vi "Odometry.vi"() -> ()   [LabVIEW 2019]
uses:
  <vilib>/myRIO/Common/Instrument Driver Framework/myRIO v1.0/Encoder/typedefs/Encoder Signal Mode.ctl
  <vilib>/myRIO/Instrument Drivers/Onboard IO/Encoder/typedefs/Encoder Reference.ctl
  <vilib>/myRIO/Common/Instrument Driver Framework/Utilities/typedefs/myRIO Generic Hardware Reference.ctl
  <vilib>/myRIO/Common/Instrument Driver Framework/Utilities/typedefs/Hardware Version Enum.ctl
  <vilib>/myRIO/Common/Instrument Driver Framework/Utilities/typedefs/myRIO v1.0 Reference.ctl
  <vilib>/myRIO/Common/Instrument Driver Framework/Utilities/typedefs/Generic FPGA Reference.ctl
  <vilib>/myRIO/Common/Instrument Driver Framework/myRIO v1.0/Encoder/typedefs/Encoder Channels Enum.ctl
  <vilib>/myRIO/Common/Instrument Driver Framework/myRIO v1.0/Encoder/typedefs/Encoder Configuration v1.0.ctl
  <vilib>/userDefined/High Color/nirio_resource_hc.ctl
  <vilib>/Platform/TimedLoop/XDataNode/timing_clust.ctl
  <vilib>/Platform/TimedLoop/XDataNode/nitl_modes.ctl
  <vilib>/Platform/TimedLoop/XDataNode/wakeup.ctl
  <vilib>/myRIO/Instrument Drivers/Onboard IO/PWM/typedefs/PWM Reference.ctl
  <vilib>/myRIO/Common/Instrument Driver Framework/myRIO v1.0/PWM/typedefs/PWM Channels Enum.ctl
  <vilib>/myRIO/Instrument Drivers/Onboard IO/PWM/typedefs/PWM Configuration.ctl
  <vilib>/myRIO/Instrument Drivers/Onboard IO/DIO/typedefs/DIO Reference.ctl
  <vilib>/myRIO/Common/Instrument Driver Framework/myRIO v1.0/DIO/typedefs/DIO Channels List.ctl
  <vilib>/myRIO/Common/Instrument Driver Framework/myRIO v1.0/DIO/typedefs/DIO Channels Enum.ctl
  <vilib>/myRIO/Common/Instrument Driver Framework/Utilities/vis/Is FPGA Ref Available.vi
  <vilib>/myRIO/Common/Instrument Driver Framework/myRIO v1.0/Encoder/vis/myRIO v1.1 Open Encoder.vi
  <vilib>/myRIO/Instrument Drivers/Onboard IO/Encoder/vis/Read.vi
  <vilib>/myRIO/Common/Instrument Driver Framework/myRIO v1.0/PWM/vis/myRIO v1.1 Open PWM.vi
  <vilib>/myRIO/Instrument Drivers/Onboard IO/PWM/vis/Set Duty Cycle and Frequency.vi
  <vilib>/myRIO/Common/Instrument Driver Framework/myRIO v1.0/DIO/vis/myRIO v1.1 Open DIO.vi
  <vilib>/myRIO/Instrument Drivers/Onboard IO/DIO/vis/Write.vi
  <vilib>/myRIO/Common/Instrument Driver Framework/Utilities/vis/Validate Channels.vi
  <vilib>/myRIO/Common/Instrument Driver Framework/myRIO v1.0/Encoder/vis/myRIO v1.0 Reserve Encoder.vi
  <vilib>/myRIO/Common/Instrument Driver Framework/myRIO v1.0/PWM/vis/myRIO v1.0 Reserve PWM.vi
  <vilib>/myRIO/Common/Instrument Driver Framework/myRIO v1.0/DIO/vis/myRIO v1.0 Reserve DIO.vi
  <vilib>/myRIO/Common/Instrument Driver Framework/myRIO v1.0/Encoder/vis/myRIO v1.0 Build MUX Configuration Encoder.vi
  <vilib>/myRIO/Common/Instrument Driver Framework/myRIO v1.0/Resource Manager/vis/myRIO v1.0 Reserve Channel List.vi
  <vilib>/myRIO/Common/Instrument Driver Framework/myRIO v1.0/PWM/vis/myRIO v1.0 Build MUX Configuration PWM.vi
  <vilib>/myRIO/Common/Instrument Driver Framework/myRIO v1.0/DIO/vis/myRIO v1.0 Build MUX Configuration DIO.vi
  <vilib>/myRIO/Common/Instrument Driver Framework/myRIO v1.0/Resource Manager/vis/myRIO v1.0 Create Configuration List.vi
  <vilib>/myRIO/Common/Instrument Driver Framework/myRIO v1.0/Resource Manager/vis/myRIO v1.0 Reserve Channel.vi
  <vilib>/myRIO/Common/Instrument Driver Framework/myRIO v1.0/Resource Manager/vis/myRIO v1.0 Unreserve Channel.vi
  <vilib>/myRIO/Common/Instrument Driver Framework/myRIO v1.0/Resource Manager/vis/myRIO v1.0 Build Mutex Name.vi
  <vilib>/Utility/VariantDataType/GetNumericInfo.vi
  <vilib>/Utility/error.llb/Error Cluster From Error Code.vi
  <vilib>/myRIO/Common/Instrument Driver Framework/myRIO v1.0/myRIO v1.1 Open.vi
  <vilib>/myRIO/Common/Instrument Driver Framework/Utilities/vis/IO Manager.vi
  <vilib>/myRIO/Common/Instrument Driver Framework/Utilities/vis/Configuration Manager.vi
  <vilib>/myRIO/Common/Instrument Driver Framework/myRIO v1.0/Resource Manager/vis/myRIO v1.0 Configure IO.vi
  <vilib>/myRIO/Common/Instrument Driver Framework/myRIO v1.0/myRIO v1.0 Close.vi
  <vilib>/myRIO/Common/Instrument Driver Framework/myRIO v1.0/Encoder/vis/myRIO v1.0 Configure Encoder.vi
  <vilib>/myRIO/Common/Instrument Driver Framework/myRIO v1.0/Encoder/vis/myRIO v1.0 Read Encoder.vi
  <vilib>/imath/engines/lvmath2/RunTimeEngine/NodeEndStatement/NIMS_NodeEndStatement_Output.vi
  <instcachedir>/0/NIMS_NodeEndStatement_Output_53EC0D466D134D7ABD903AC30B43404B.lvgen/NIMS_NodeEndStatement_Output_53EC0D466D134D7ABD903AC30B43404B_001.vi
  <vilib>/imath/engines/lvmath2/RunTimeEngine/ErrorHandling/NIMS_Finalize Error.vi
  <vilib>/myRIO/Common/Instrument Driver Framework/myRIO v1.0/PWM/vis/myRIO v1.0 Write PWM.vi
  <vilib>/myRIO/Common/Instrument Driver Framework/myRIO v1.0/DIO/vis/myRIO v1.0 Write DIO.vi
  <vilib>/imath/engines/lvmath2/RunTimeEngine/Managers/WorkSpace/UID Generator.vi
  <vilib>/imath/engines/lvmath2/RunTimeEngine/RunTimeType/NIMS_RunTimeType_From StrictType (excl LVString).vi
  <instcachedir>/0/NIMS_RunTimeType_From StrictType (excl LVString)_D8AFBA86A94845AAA577C895450664BD.lvgen/NIMS_RunTimeType_From StrictType (excl LVString)_D8AFBA86A94845AAA577C895450664BD_000.vi
  <vilib>/imath/engines/lvmath2/RunTimeEngine/LocalVariableDefStatement/MC_LocalVariableDefStatement_Display.vi
  <vilib>/imath/engines/lvmath2/RunTimeEngine/Managers/SymbolTable/Clear UID.vi
  <vilib>/myRIO/Express VI/Onboard IO/Encoder/Encoder Express VI.xnode
  <vilib>/myRIO/Instrument Drivers/Onboard IO/Encoder/vis/myRIO Encoder Open.xnode
  <vilib>/myRIO/Common/Instrument Driver Framework/myRIO v1.0/Encoder/typedefs/Encoder Count Direction Enum.ctl
  <vilib>/platform/TimedLoop/XDataNode/XDataNode.xnode
  <vilib>/myRIO/Express VI/Onboard IO/PWM/PWM Express VI.xnode
  <vilib>/myRIO/Instrument Drivers/Onboard IO/PWM/vis/myRIO PWM Open.xnode
  <vilib>/myRIO/Express VI/Onboard IO/DO/DO Express VI.xnode
  <vilib>/myRIO/Instrument Drivers/Onboard IO/DIO/vis/myRIO DIO Open.xnode
  <vilib>/Platform/TimedLoop/XDataNode/XDNodeRunTimeDep.lvlib
  <vilib>/myRIO/Instrument Drivers/Onboard IO/DIO/DIO.lvlib
  <vilib>/myRIO/Instrument Drivers/Onboard IO/Encoder/Encoder.lvlib
  <vilib>/myRIO/Instrument Drivers/Onboard IO/PWM/PWM.lvlib
  <vilib>/imath/engines/lvmath2/RunTimeEngine/Managers/SymbolTable/NIMS_WorkSpace.lvlib
panel:
  out "phiR chart case1":dynamicdata(graph)
  out "omegaR chart case1":dynamicdata(graph)
  in  "Tab Control":enum32{"Page 1", "Page 2", "Page 3"}(tab)
  out "XY Graph":cluster{"X":dbl, "Y":dbl}[](graph)
  in  "t1":dbl
  in  "t2":dbl
  in  "t3":dbl
  in  "Vmax (m/s)":dbl
  out "omega R now, desired case1":cluster{dbl, "omegaR":dbl}(graph)
  out "CarOmega case1":cluster{"actCarOmega":dbl, "desCarOmega":dbl}(graph)
  out "CarV case1":cluster{"actCarV":dbl, "desCarV":dbl}(graph)
  out "omega L now, desired case1":cluster{dbl, "omegaL":dbl}(graph)
  out "carV chart case1":dynamicdata(graph)
  out "omegaR":dbl
  out "omegaL":dbl
  in  "Stop case1":bool
  in  "Frequency R [Hz] case1":dbl=1000.0
  out "Duty R case1":dbl
  out "Duty L case1":dbl
  in  "Frequency L [Hz] case1":dbl=1000.0
  out "phiR":dbl
  out "phiL":dbl
  in  "R Gain":T1
  in  "L Gain":T1
  out "Encoder R":i32
  out "desPhiR":dbl
  out "CarOmega case2":cluster{"actCarOmega":dbl, "desCarOmega":dbl}(graph)
  out "CarV case2":cluster{"actCarV":dbl, "desCarV":dbl}(graph)
  in  "t5 case2":dbl
  in  "t6 case2":dbl
  in  "t7 case2":dbl
  in  "t8 case2":dbl
  in  "t9 case2":dbl
  in  "stop case2":bool
  in  "t4 case2":dbl
  out "Duty L case2":dbl
  in  "Frequency L [Hz] case2":dbl=1000.0
  out "phi L now, desired case2":cluster{dbl, "omegaL":dbl}(graph)
  out "phi R now, desired case2":cluster{dbl, "omegaR":dbl}(graph)
  in  "Vmax (m/s) case2":dbl
  in  "t1 case2":dbl
  in  "t2 case2":dbl
  in  "t3 case2":dbl
  in  "thetaDotmax case2":dbl
  out "carVTest Chart case2":dynamicdata(graph)
  out "XY Graph case2":dbl[][](graph)
  out "thetaDot case2":dbl
  out "carOmegaTest case2":dynamicdata(graph)
  in  "Frequency R [Hz] case2":dbl=1000.0
  out "Duty R case2":dbl
  in  "R Gain case2":T1
  in  "L Gain case2":T1
  in  "thetaDotmax case3":dbl
  in  "t7 case3":dbl
  in  "t6 case3":dbl
  in  "t5 case3":dbl
  in  "t4 case3":dbl
  in  "t3 case3":dbl
  in  "t2 case3":dbl
  in  "t1 case3":dbl
  out "thetaDot case3":dbl
  in  "Vmax (m/s) case3":dbl
  in  "stop case3":bool
  out "Duty R case3":dbl
  in  "Frequency R [Hz] case3":dbl=1000.0
  in  "Frequency L [Hz] case3":dbl=1000.0
  out "Duty L case3":dbl
  out "XY Graph case3":dbl[][](graph)
  out "phi L now, desired case3":cluster{dbl, "omegaL":dbl}(graph)
  out "CarV case3":cluster{"actCarV":dbl, "desCarV":dbl}(graph)
  out "CarOmega case3":cluster{"actCarOmega":dbl, "desCarOmega":dbl}(graph)
  out "phi R now, desired case3":cluster{dbl, "omegaR":dbl}(graph)
  out "carV Chart case3":dynamicdata(graph)
  out "carOmega Chart case3":dynamicdata(graph)
  in  "R Gain case3":T1
  in  "L Gain case3":T1
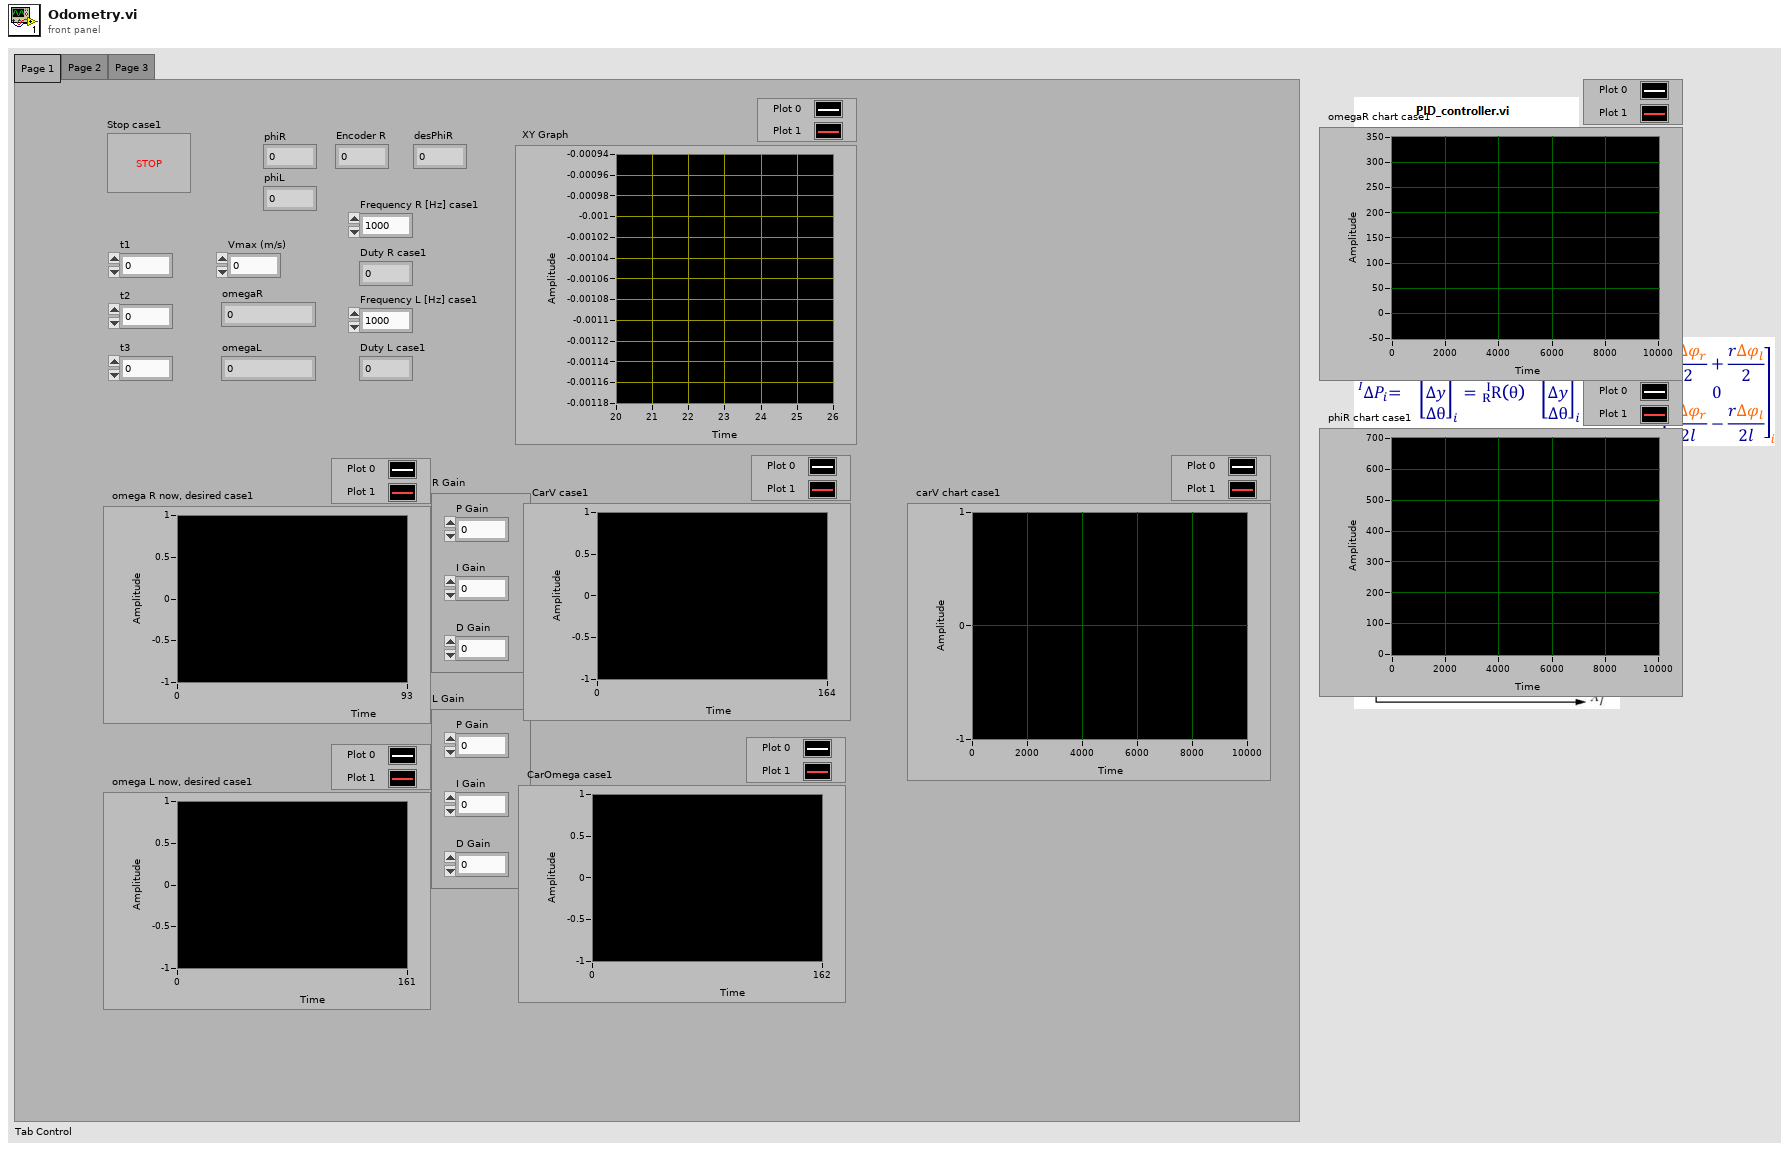
[diagram p1: front panel]
types:
  T1 = cluster{"P Gain":dbl, "I Gain":dbl, "D Gain":dbl}
  T2 = typedef "Encoder.lvlib/Encoder Reference.ctl" = cluster{"myRIO Reference":T3, "Encoder Channels Enum":T7}
  T3 = typedef "myRIO Generic Hardware Reference.ctl" = cluster{"myRIO Model":T4, "myRIO Hardware Reference":T5}
  T4 = typedef "Hardware Version Enum.ctl" = enum16{"Unknown", "myRIO-1900", "myRIO-1950", "roboRIO", "NI ELVIS RIO CM", "ELVIS III"}
  T5 = typedef "myRIO v1.0 Reference.ctl" = cluster{"Generic FPGA Reference":T6, "Allow multiple opens":bool}
  T6 = typedef "Generic FPGA Reference.ctl" = refnum<k20>
  T7 = typedef "Encoder Channels Enum.ctl" = enum16{"Not Connected", "C/ENC0", "C/ENC1", "A/ENC", "A/ENC0", "A/ENC1", "A/ENC2", "A/ENC3", "A/ENC4", "A/ENC5", "A/ENC6", "A/ENC7", "A/ENC8", "A/ENC9", "B/ENC", "B/ENC0", "B/ENC1", "B/ENC2", "B/ENC3", "B/ENC4", "B/ENC5", "B/ENC6", "B/ENC7", "B/ENC8", "B/ENC9", "DIO/ENC0", "DIO/ENC1", "DIO/ENC2", "DIO/ENC3", "DIO/ENC4"}
  T8 = typedef "Encoder Signal Mode.ctl" = enum16{"Quadrature phase signal", "Step and direction signal"}
  T9 = typedef "nirio_resource_hc.ctl" = tag
  T10 = typedef "PWM.lvlib/PWM Reference.ctl" = cluster{"myRIO Reference":T3, "PWM Channels Enum":T11, "PWM Configuration":T12}
  T11 = typedef "PWM Channels Enum.ctl" = enum16{"Not Connected", "C/PWM0", "C/PWM1", "A/PWM0", "A/PWM1", "A/PWM2", "A/PWM3", "A/PWM4", "A/PWM5", "A/PWM6", "A/PWM7", "A/PWM8", "A/PWM9", "A/PWM10", "A/PWM11", "A/PWM12", "A/PWM13", "A/PWM14", "A/PWM15", "A/PWM16", "A/PWM17", "A/PWM18", "A/PWM19", "B/PWM0", "B/PWM1", "B/PWM2", "B/PWM3", "B/PWM4", "B/PWM5", "B/PWM6", "B/PWM7", "B/PWM8", "B/PWM9", "B/PWM10", "B/PWM11", "B/PWM12", "B/PWM13", "B/PWM14", "B/PWM15", "B/PWM16", "B/PWM17", "B/PWM18", "B/PWM19", "PWM/PWM0", "PWM/PWM1", "PWM/PWM2", "PWM/PWM3", "PWM/PWM4", "PWM/PWM5", "PWM/PWM6", "PWM/PWM7", "PWM/PWM8", "PWM/PWM9"}
  T12 = typedef "PWM.lvlib/PWM Configuration.ctl" = cluster{"Frequency":dbl, "Duty Cycle":dbl}
  T13 = typedef "DIO.lvlib/DIO Reference.ctl" = cluster{"myRIO Reference":T3, "DIO Channels List":T14}
  T14 = typedef "DIO Channels List.ctl" = T15[]
  T15 = typedef "DIO Channels Enum.ctl" = enum16{"Not Connected", "C/DIO0", "C/DIO1", "C/DIO2", "C/DIO3", "C/DIO4", "C/DIO5", "C/DIO6", "C/DIO7", "A/DIO0", "A/DIO1", "A/DIO2", "A/DIO3", "A/DIO4", "A/DIO5", "A/DIO6", "A/DIO7", "A/DIO8", "A/DIO9", "A/DIO10", "A/DIO11", "A/DIO12", "A/DIO13", "A/DIO14", "A/DIO15", "A/DIO16", "A/DIO17", "A/DIO18", "A/DIO19", "B/DIO0", "B/DIO1", "B/DIO2", "B/DIO3", "B/DIO4", "B/DIO5", "B/DIO6", "B/DIO7", "B/DIO8", "B/DIO9", "B/DIO10", "B/DIO11", "B/DIO12", "B/DIO13", "B/DIO14", "B/DIO15", "B/DIO16", "B/DIO17", "B/DIO18", "B/DIO19", "LED0", "LED1", "LED2", "LED3", "Button0", "DIO/DIO0", "DIO/DIO1", "DIO/DIO2", "DIO/DIO3", "DIO/DIO4", "DIO/DIO5", "DIO/DIO6", "DIO/DIO7", "DIO/DIO8", "DIO/DIO9", "SPI/CS0", "SPI/CS1", "SPI/CS2", "SPI/CS3", "LED RADIO (Green)", "LED RADIO (Red)", "LED COMM (Green)", "LED COMM (Red)", "LED MODE (Green)", "LED MODE (Red)"}
  T16 = typedef "XDNodeRunTimeDep.lvlib/timing_clust.ctl" = cluster{"Expected End [f-1]":u64, "Actual End [f-1]":u64, "Finished Late? [f-1]":bool, "Expected End [i-1]":u64, "Actual End [i-1]":u64, "Finished Late? [i-1]":bool, "Expected Start [i]":u64, "Actual Start [i]":u64, "Expected Start [f]":u64, "Actual Start [f]":u64, "Source Name":string, "Structure Name":string, "Period":i64, "Deadline":i64, "Offset":i64, "Start":i64, "Priority":i32, "Timeout":i32, "Mode":T17, "Wakeup Reason":T18, "Error":errorcluster, "Source Type":string, "Secondary Source Type":string, "Global End Time":u64, "Global Start Time":u64, "Frame Duration":u64, "Iteration Duration":u64, "Assigned CPU":i32, "I/O Scan Engine Mode":u32}
  T17 = typedef "XDNodeRunTimeDep.lvlib/nitl_modes.ctl" = enum32{"No Change", "Process missed periods, maintain original phase", "Discard missed periods, maintain original phase", "Process missed periods, ignore original phase", "Discard missed periods, ignore original phase"}
  T18 = typedef "XDNodeRunTimeDep.lvlib/wakeup.ctl" = enum32{"Normal", "Aborted", "Asynchronous wakeup", "Timing source error", "Timed loop error", "Timeout"}
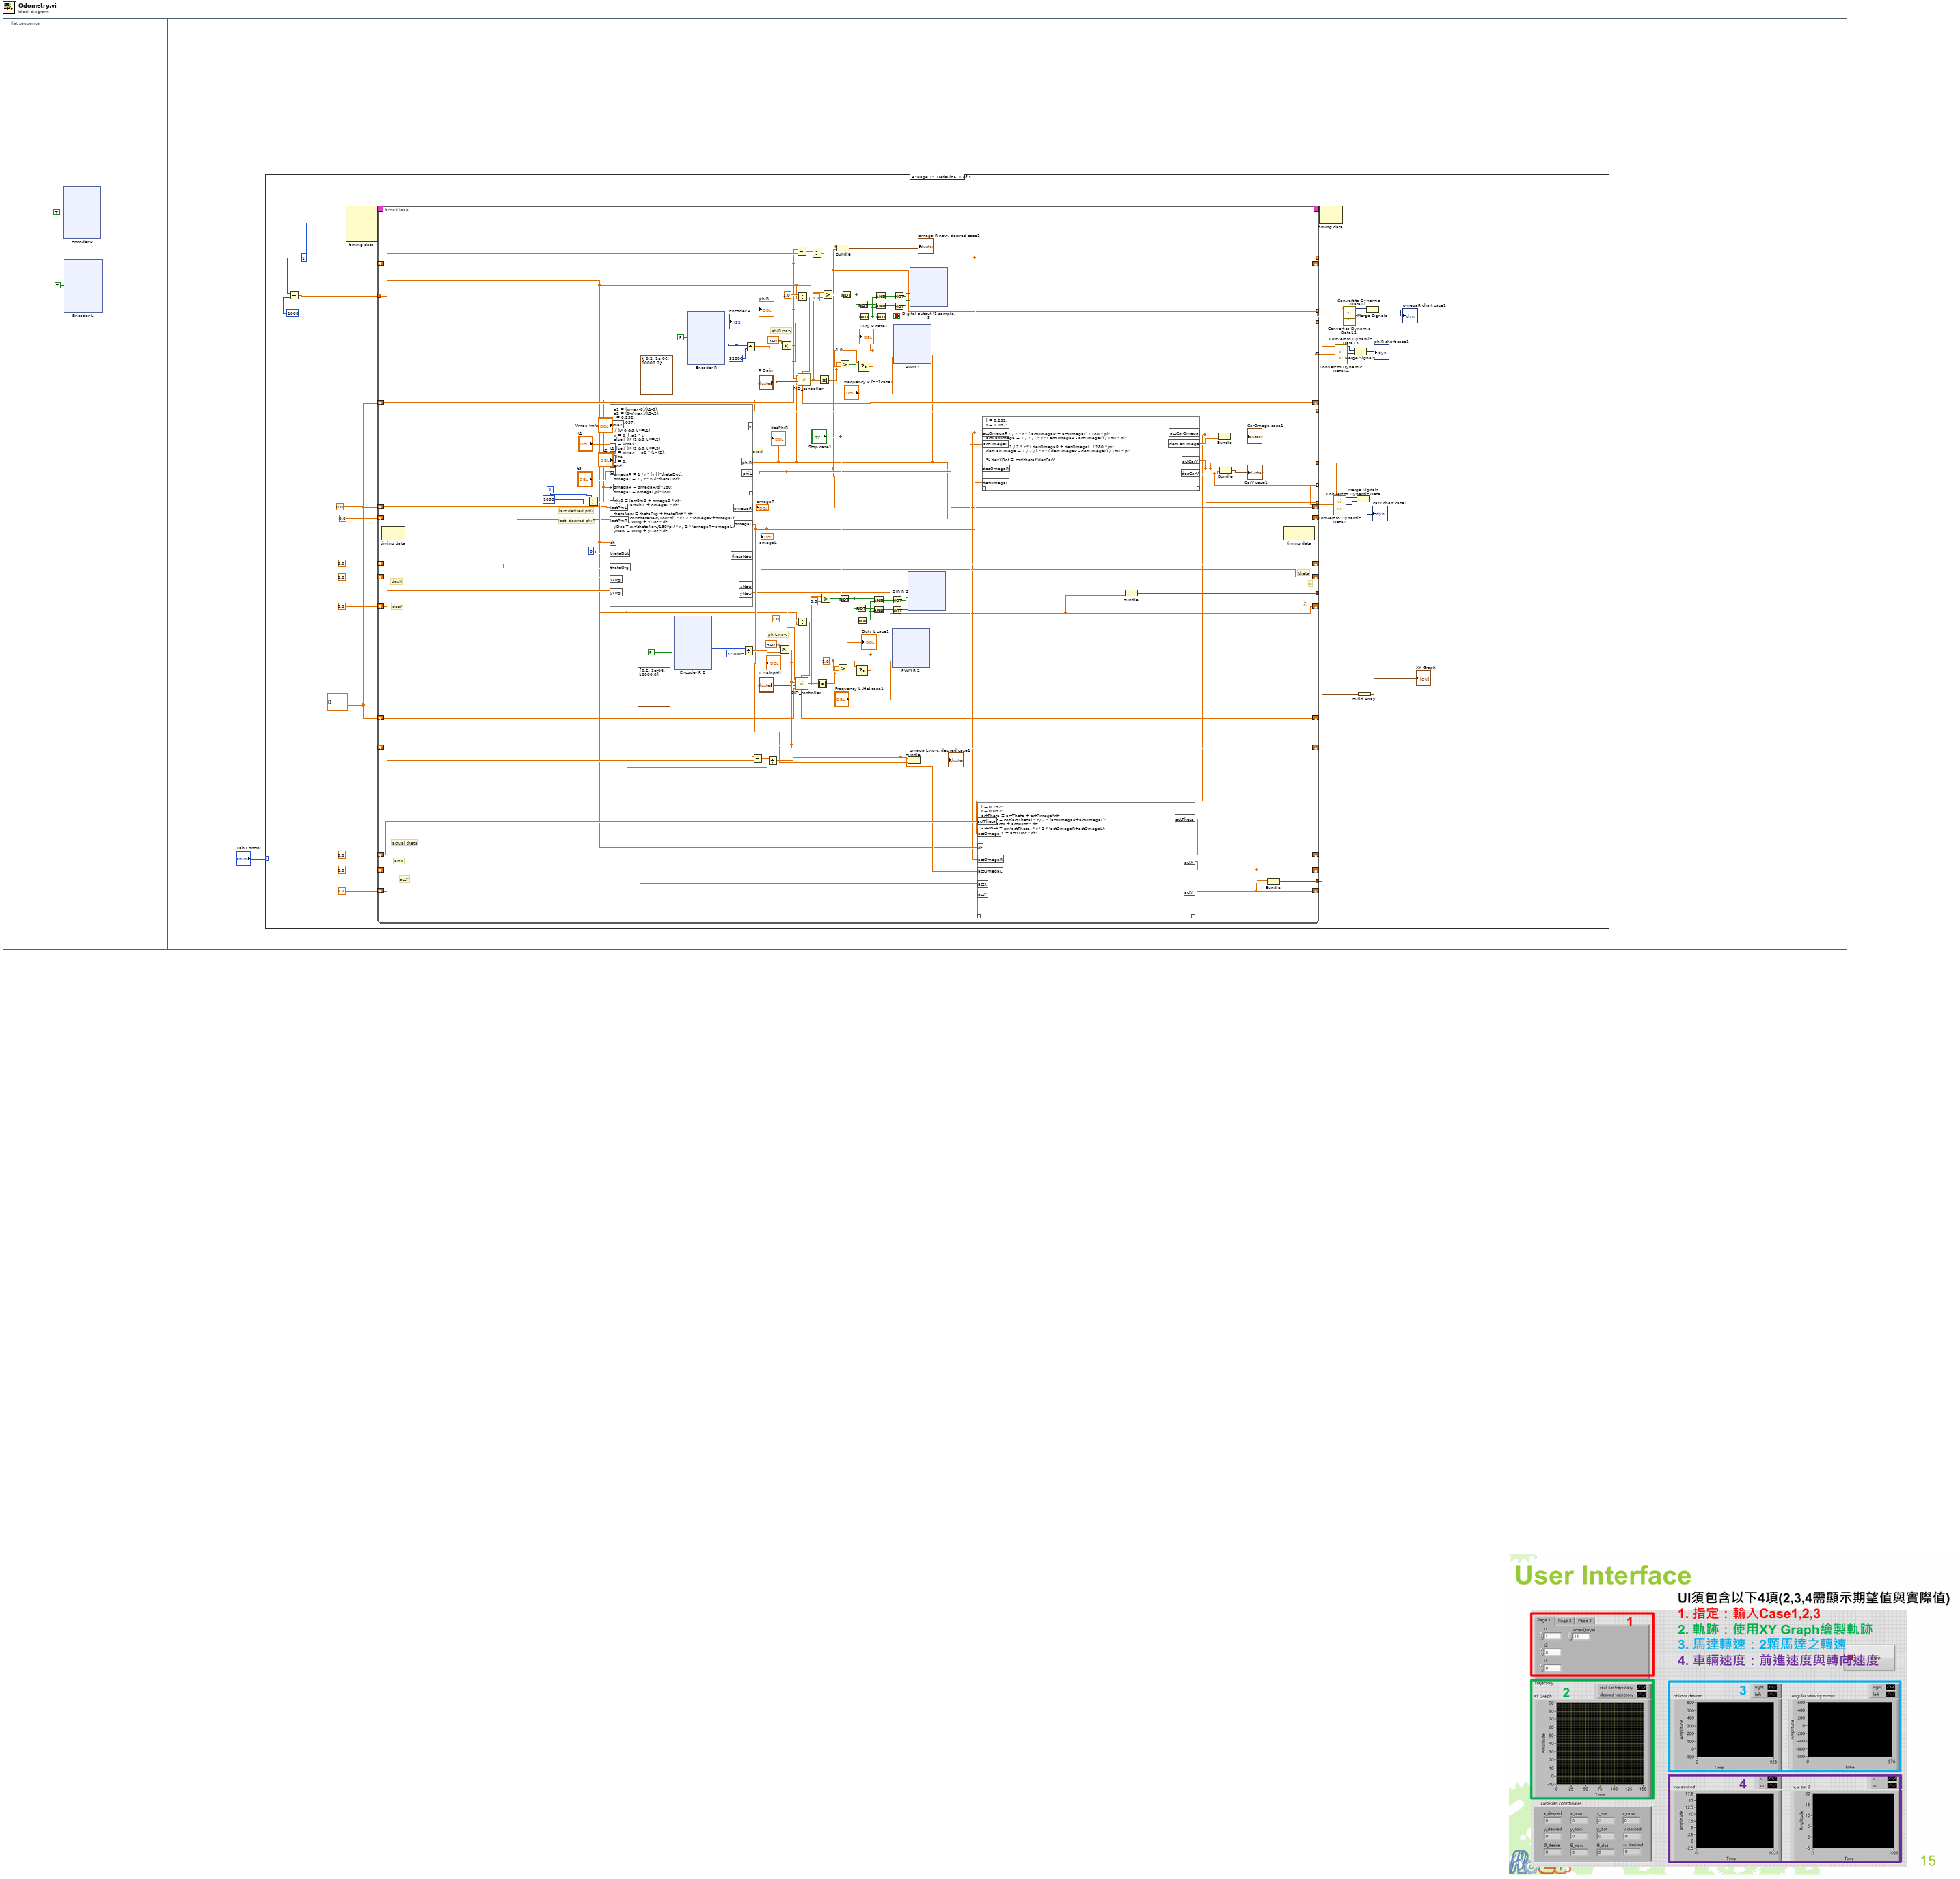
[diagram p0: block diagram]
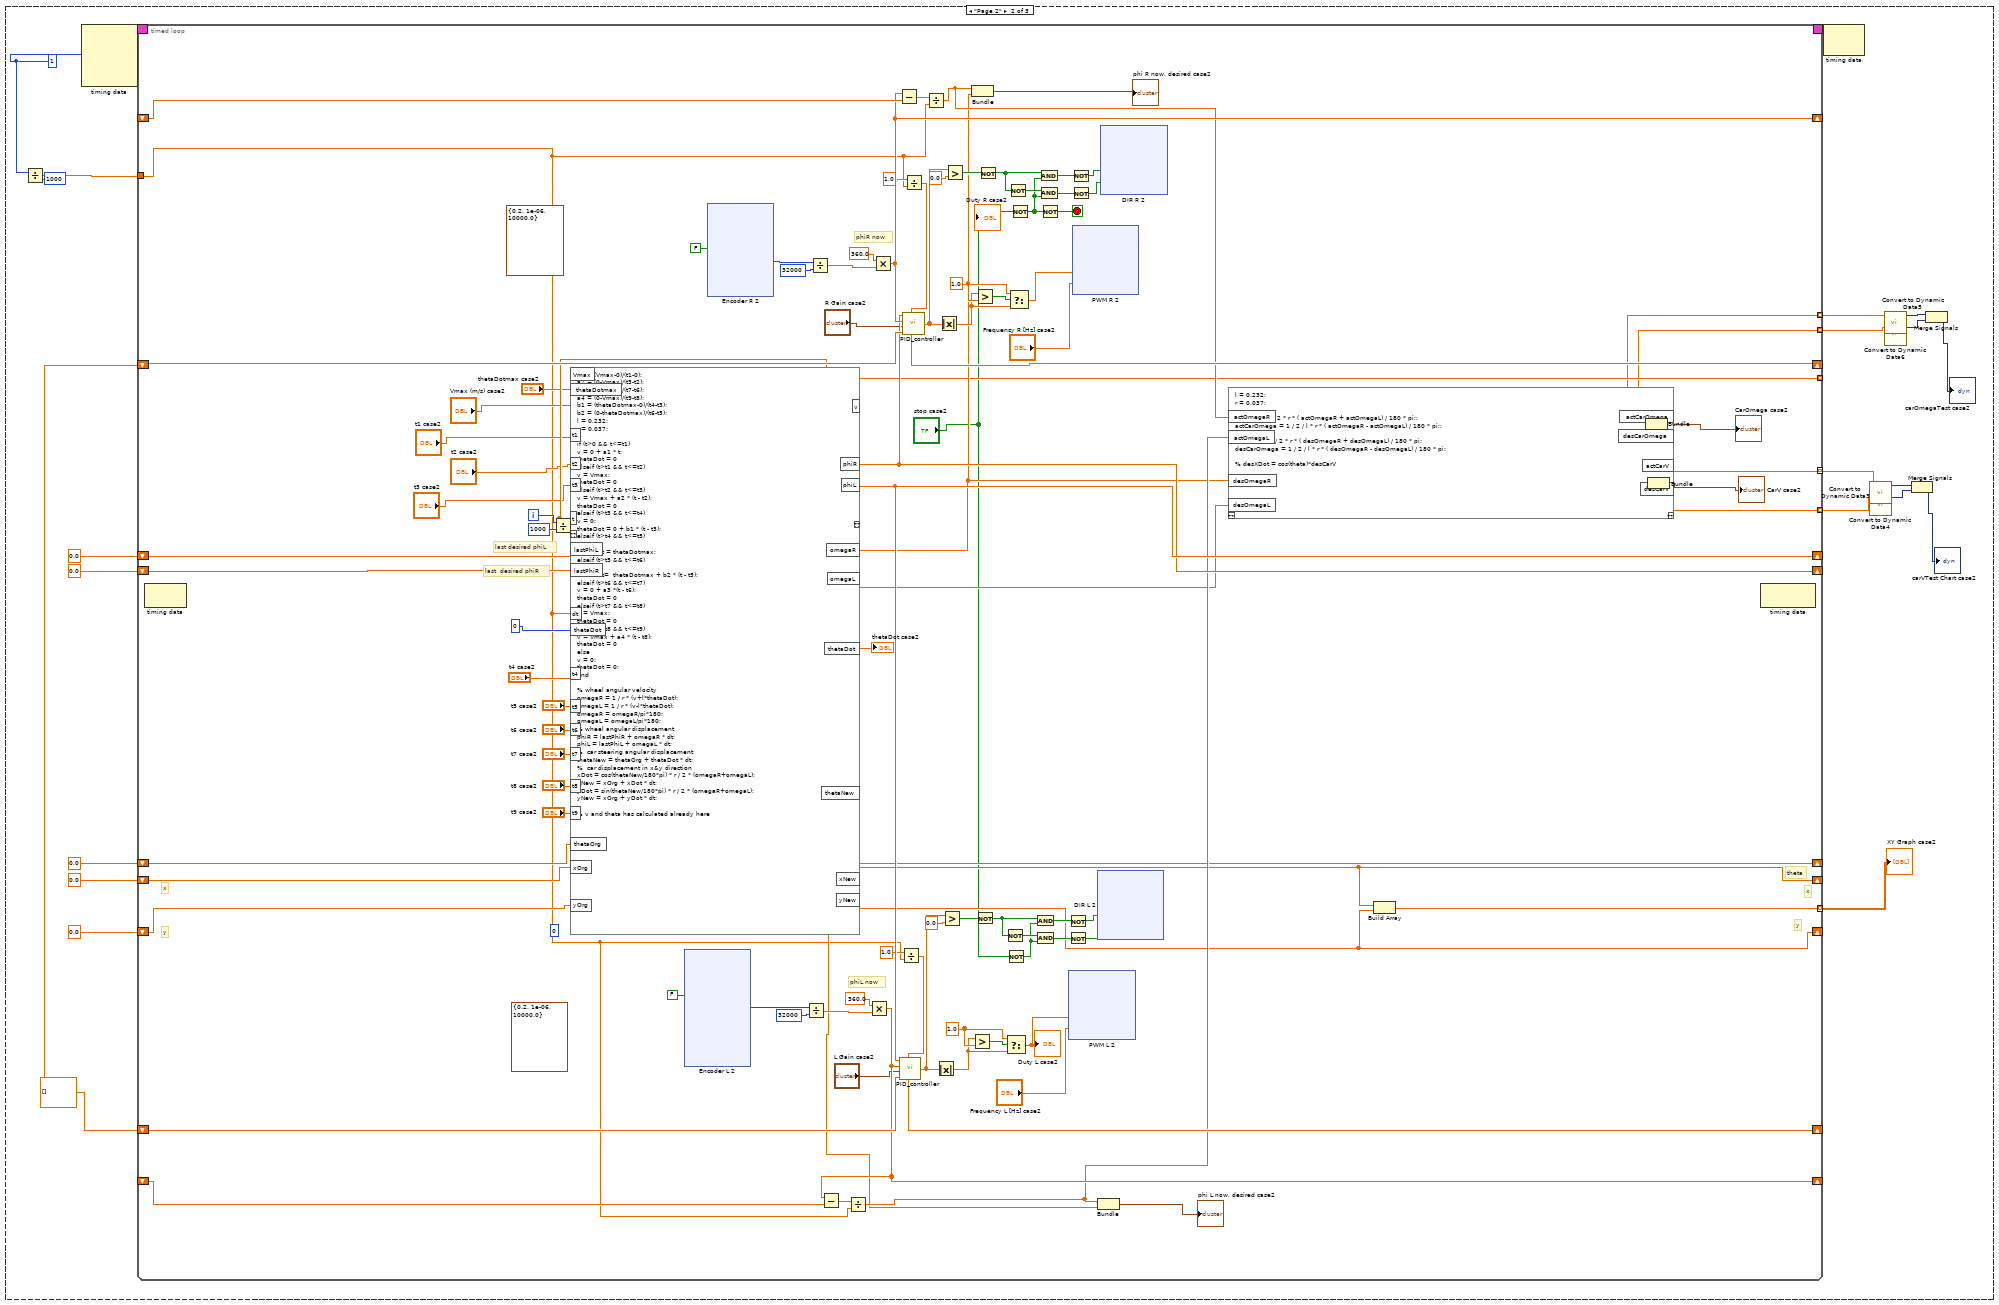
[diagram p2: hidden frame]
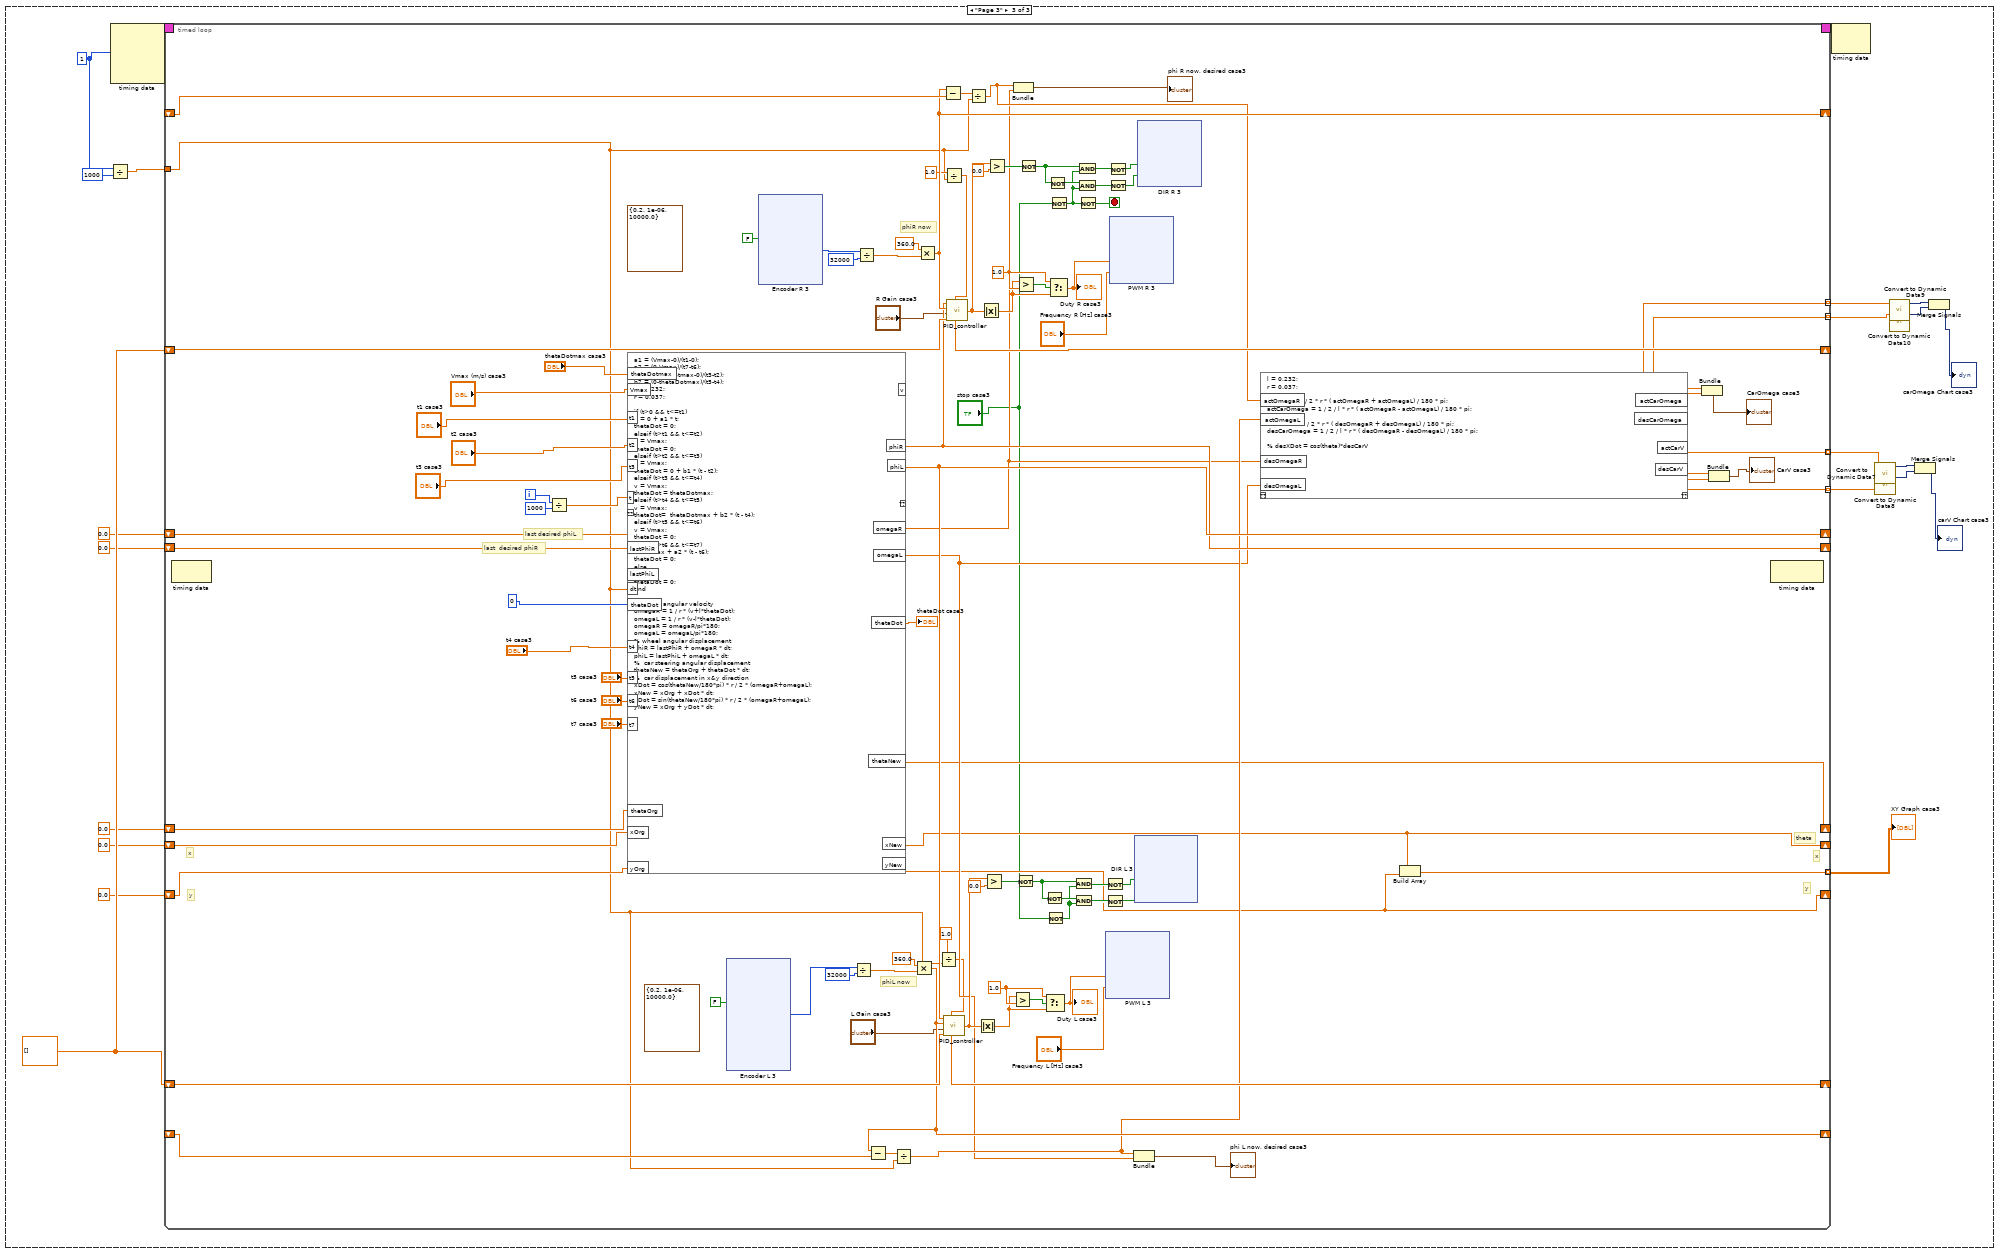
[diagram p3: hidden frame]
diagram:
  n1 = flat-sequence {
    frame #0 {
      n2 = xnode "Encoder R"("Reset Counter"=TRUE) -> ()  [unwired: 1 in, 4 out]
      n3 = xnode "Encoder L"("Reset Counter"=TRUE) -> ()  [unwired: 1 in, 4 out]
    }
    frame #1 {
      n4 = case shown="\"Page 1\", Default" "Tab Control" {
        frame "Page 1", Default {
          w119 = dbl[] [] ("state(k)")
          w118 = i64 1 ("Period")
          n5 = Divide(x=w118, y=i64 1000) -> (x/y=w106:dbl)
          n6 = node-c288(w118) -> (w126:T16)  [unwired: 3 in]
          n7 = timed-loop {
            timing: w126 -> [_]
            timing-out: [_] -> w125
            shift-right: [w128] -> _
            shift-left: 0.0 ("phiR") -> [w130]
            shift-right: [w138] -> _
            shift-left: 0.0 ("phiL") -> [w129]
            tunnel: w106 -> [w133]
            shift-right: [w213] -> _
            shift-left: w119 -> [w214]
            shift-right: [w182] -> _
            shift-left: w119 -> [w181]
            shift-right: [w127] -> _
            shift-left: _ -> [w179]
            shift-right: [w174] -> _
            shift-left: _ -> [w175]
            shift-right: [w168] -> _
            shift-left: 0.0 ("thetaNew") -> [w161]
            shift-right: [w151] -> _
            shift-left: 0.0 ("xNew") -> [w167]
            shift-right: [w150] -> _
            shift-left: 0.0 ("yNew") -> [w166]
            tunnel: [w164] -> _ mode=indexing
            tunnel: [w162] -> _ mode=indexing
            tunnel: [w163] -> w123 mode=indexing
            tunnel: [w162] -> w124 mode=indexing
            shift-right: [w152] -> _
            shift-left: 0.0 ("actTheta") -> [w157]
            shift-right: [w148] -> _
            shift-left: 0.0 ("actX") -> [w154]
            shift-right: [w147] -> _
            shift-left: 0.0 ("actY") -> [w153]
            tunnel: [w149] -> _
            tunnel: [w146] -> w97
            tunnel: [w132] -> w113 mode=indexing
            tunnel: [w131] -> w112 mode=indexing
            tunnel: [w127] -> w111 mode=indexing
            tunnel: [w128] -> w110 mode=indexing
            i -> [w220]
            stop <- w205 stop-if-true
            w185 = 1.0 ("y")
            (unwired) cluster{dbl, dbl, dbl} {0.2, 1e-06, 10000.0}
            w203 = 1.0 ("y")
            (unwired) cluster{dbl, dbl, dbl} {-0.2, 1e-06, 10000.0}
            # "actY"
            # "actX"
            # "actual theta"
            # "y"
            # "desY"
            # "x"
            # "desX"
            # "theta"
            # "desired"
            # "phiL now"
            # "phiR now"
            # "last desired phiL"
            # "last  desired phiR"
            n8 = node-c288() -> ()  [unwired: 1 in, 1 out]
            n9 = Divide(x=w220, y=1000) -> (x/y=w164:dbl)
            n10 = mathscript code="a1 = (Vmax-0)/(t1-0);\na2 = (0-Vmax)/(t3-t2);\nl = 0.232;\nr = 0.037;\n\nif (t>0 && t<=t1)\nv = 0 + a1 * t;\nelseif (t>t1 && t<=t2)\nv = Vmax;\nelseif (t>t2 && t<=t3)\nv = Vmax + a2 * (t - t2);\nelse\nv = 0;\nend\n\nomegaR = 1 / r * (v+l*thetaDot);\nomegaL = 1 / r * (v-l*thetaDot);\n\nomegaR = omegaR/pi*180;\nomegaL = omegaL/pi*180;\n\nphiR = lastPhiR + omegaR * dt;\nphiL = lastPhiL + omegaL * dt;\n\nthetaNew = thetaOrg + thetaDot * dt;\nxDot = cos(thetaNew/180*pi) * r / 2 * (omegaR+omegaL);\nxNew = xOrg + xDot * dt;\nyDot = sin(thetaNew/180*pi) * r / 2 * (omegaR+omegaL);\nyNew = xOrg + yDot * dt;"("t1"="t1", "t2"="t2", "t3"="t3", "Vmax"="Vmax (m/s)", "t"=w164, "lastPhiR"=w130, "lastPhiL"=w129, "dt"=w133, "thetaDot"=0, "thetaOrg"=w161, "xOrg"=w167, "yOrg"=w166) -> ("omegaR"=w131:dbl, "omegaL"=w172:dbl, "phiL"=w138:dbl, "phiR"=w128:dbl, "thetaNew"=w168:dbl, "xNew"=w151:dbl, "yNew"=w150:dbl)  [unwired: 1 in, 2 out]
            "omegaR" <- w131
            "omegaL" <- w172
            "desPhiR" <- w128
            n11 = xnode "Encoder R 2"("Reset Counter"=FALSE) -> ("Counter Value"=w198:i32)  [unwired: 1 in, 3 out]
            n12 = xnode "Encoder R"("Reset Counter"=FALSE) -> ("Counter Value"=w217:i32)  [unwired: 1 in, 3 out]
            "Encoder R" <- w217
            n13 = Divide(x=w198, y=32000) -> (x/y=w199:dbl)
            n14 = Divide(x=w217, y=32000) -> (x/y=w218:dbl)
            n15 = Multiply(x=360.0, y=w199) -> (x*y=w174:dbl)
            "phiL" <- w174
            n16 = Subtract(x=w174, y=w175) -> (x-y=w176:dbl)
            n17 = Divide(x=w176, y=w133) -> (x/y=w155:dbl)
            n18 = Multiply(x=360.0, y=w218) -> (x*y=w127:dbl)
            "phiR" <- w127
            n19 = Subtract(x=w127, y=w179) -> (x-y=w178:dbl)
            n20 = Divide(x=1.0 ("y"), y=w133) -> (x/y=w137:dbl)
            n21 = Divide(x=1.0 ("y"), y=w133) -> (x/y=w136:dbl)
            n22 = call "PID_controller.vi"("Time Period"=w136, "state(k-1)"=w181, "Gain"="L Gain", "variable"=w174, "set point"=w138) -> ("PID gain"=w183:dbl, "state(k)"=w182:dbl[])
            n23 = call "PID_controller.vi"("Time Period"=w137, "state(k-1)"=w214, "Gain"="R Gain", "variable"=w127, "set point"=w128) -> ("PID gain"=w201:dbl, "state(k)"=w213:dbl[])
            n24 = Divide(x=w178, y=w133) -> (x/y=w132:dbl)
            n25 = Absolute Value(x=w183) -> (abs(x)=w184:dbl)
            n26 = Absolute Value(x=w201) -> (abs(x)=w202:dbl)
            n27 = Greater?(x=w183, y=0.0) -> (0:w190:bool)
            n28 = Greater?(x=w201, y=0.0) -> (0:w209:bool)
            n29 = Greater?(x=w184, y=w185) -> (0:w186:bool)
            n30 = Bundle(w132, "omegaR"=w131) -> (→"omega R now, desired case1":cluster{dbl, "omegaR":dbl})  [unwired: 1 in]
            n31 = Not(x=w190) -> (.not. x?=w191:bool)
            n32 = Greater?(x=w202, y=w203) -> (0:w204:bool)
            n33 = Not(x=w209) -> (.not. x?=w210:bool)
            n34 = Not(x=w191) -> (.not. x?=w188:bool)
            n35 = Select(t=w185, s=w186, f=w184) -> (s? t:f=w158:dbl)
            "Duty L case1" <- w158
            n36 = Not(x="Stop case1") -> (.not. x?=w187:bool)
            n37 = Not(x=w210) -> (.not. x?=w207:bool)
            n38 = Select(t=w203, s=w204, f=w202) -> (s? t:f=w143:dbl)
            "Duty R case1" <- w143
            n39 = Not(x="Stop case1") -> (.not. x?=w206:bool)
            n40 = And(x=w191, y=w187) -> (x .and. y?=w194:bool)
            n41 = And(x=w188, y=w187) -> (x .and. y?=w192:bool)
            n42 = And(x=w210, y=w206) -> (x .and. y?=w212:bool)
            n43 = And(x=w207, y=w206) -> (x .and. y?=w211:bool)
            n44 = Not(x=w206) -> (.not. x?=w205:bool)
            n45 = Not(x=w194) -> (.not. x?=w195:bool)
            n46 = Not(x=w192) -> (.not. x?=w193:bool)
            n47 = xnode "PWM R 2"("Duty Cycle"=w158, "Frequency [Hz]"="Frequency L [Hz] case1") -> ()  [unwired: 1 in, 1 out]
            n48 = Not(x=w212) -> (.not. x?=w145:bool)
            n49 = Not(x=w211) -> (.not. x?=w144:bool)
            n50 = xnode "PWM 2"("Duty Cycle"=w143, "Frequency [Hz]"="Frequency R [Hz] case1") -> ()  [unwired: 1 in, 1 out]
            n51 = xnode "DIR R 2"("A/DIO0 (Pin 11)"=w195, "A/DIO1 (Pin 13)"=w193) -> ()  [unwired: 1 in, 1 out]
            n52 = Bundle(w155, "omegaL"=w172) -> (→"omega L now, desired case1":cluster{dbl, "omegaL":dbl})  [unwired: 1 in]
            n53 = xnode "Digital output (1 sample) 3"("B/DIO0 (Pin 11)"=w145, "B/DIO1 (Pin 13)"=w144) -> ()  [unwired: 1 in, 1 out]
            n54 = mathscript code="l = 0.232;\nr = 0.037;\n\nactCarV = 1 / 2 * r * ( actOmegaR + actOmegaL) / 180 * pi;\nactCarOmega = 1 / 2 / l * r * ( actOmegaR - actOmegaL) / 180 * pi;\n\ndesCarV = 1 / 2 * r * ( desOmegaR + desOmegaL) / 180 * pi;\ndesCarOmega = 1 / 2 / l * r * ( desOmegaR - desOmegaL) / 180 * pi;\n\n% desXDot = cos(theta)*desCarV"("desOmegaR"=w131, "desOmegaL"=w172, "actOmegaR"=w132, "actOmegaL"=w155) -> ("actCarOmega"=w156:dbl, "desCarOmega"=w171:dbl, "actCarV"=w162:dbl, "desCarV"=w163:dbl)  [unwired: 1 in, 1 out]
            n55 = mathscript code="l = 0.232;\nr = 0.037;\nactTheta = actTheta + actOmega*dt;\nactXDot = cos(actTheta) * r / 2 * (actOmegaR+actOmegaL);\nactX = actX + actXDot * dt;\nactYDot = sin(actTheta) * r / 2 * (actOmegaR+actOmegaL);\nactY =actY + actYDot * dt;"("actTheta"=w157, "actOmega"=w156, "dt"=w133, "actOmegaR"=w132, "actOmegaL"=w155, "actX"=w154, "actY"=w153) -> ("actTheta"=w152:dbl, "actX"=w148:dbl, "actY"=w147:dbl)  [unwired: 1 in, 1 out]
            n56 = Bundle("xNew"=w151, "yNew"=w150) -> (w149:cluster{"xNew":dbl, "yNew":dbl})  [unwired: 1 in]
            n57 = Bundle("actCarOmega"=w156, "desCarOmega"=w171) -> (→"CarOmega case1":cluster{"actCarOmega":dbl, "desCarOmega":dbl})  [unwired: 1 in]
            n58 = Bundle("actCarV"=w162, "desCarV"=w163) -> (→"CarV case1":cluster{"actCarV":dbl, "desCarV":dbl})  [unwired: 1 in]
            n59 = Bundle("actX"=w148, "actY"=w147) -> (w146:cluster{"actX":dbl, "actY":dbl})  [unwired: 1 in]
            n60 = node-c288() -> ()  [unwired: 1 in, 1 out]
          }
          n61 = node-c288(w125) -> ()  [unwired: 1 out]
          n62 = call "Convert to Dynamic Data"("Array"=w124) -> ("Dynamic Data Type"=w121:dynamicdata)  [unwired: 3 in]
          n63 = call "Convert to Dynamic Data2"("Array"=w123) -> ("Dynamic Data Type"=w120:dynamicdata)  [unwired: 3 in]
          n64 = call "Convert to Dynamic Data13"("Array"=w111) -> ("Dynamic Data Type"=w109:dynamicdata)  [unwired: 3 in]
          n65 = call "Convert to Dynamic Data14"("Array"=w110) -> ("Dynamic Data Type"=w108:dynamicdata)  [unwired: 3 in]
          n66 = call "Convert to Dynamic Data11"("Array"=w113) -> ("Dynamic Data Type"=w116:dynamicdata)  [unwired: 3 in]
          n67 = call "Convert to Dynamic Data12"("Array"=w112) -> ("Dynamic Data Type"=w115:dynamicdata)  [unwired: 3 in]
          n68 = Merge Signals(w109, w108) -> (→"phiR chart case1":dynamicdata)
          n69 = Merge Signals(w121, w120) -> (→"carV chart case1":dynamicdata)
          n70 = Build Array(w97) -> (→"XY Graph":cluster{"actX":dbl, "actY":dbl}[])
          n71 = Merge Signals(w115, w116) -> (→"omegaR chart case1":dynamicdata)
        }
        frame "Page 2" {
          w974 = dbl[] [] ("state(k)")
          w977 = i64 1 ("Period")
          n72 = Divide(x=w977, y=i64 1000) -> (x/y=w975:dbl)
          n73 = node-c288(w977) -> (w990:T16)  [unwired: 3 in]
          n74 = timed-loop {
            timing: w990 -> [_]
            timing-out: [_] -> w989
            shift-right: [w1040] -> _
            shift-left: 0.0 ("phiR") -> [w1086]
            shift-right: [w1041] -> _
            shift-left: 0.0 ("phiL") -> [w1085]
            tunnel: w975 -> [w994]
            shift-right: [w1079] -> _
            shift-left: w974 -> [w1080]
            shift-right: [w1046] -> _
            shift-left: w974 -> [w1045]
            shift-right: [w1043] -> _
            shift-left: _ -> [w1044]
            shift-right: [w1037] -> _
            shift-left: _ -> [w1038]
            shift-right: [w1022] -> _
            shift-left: 0.0 ("thetaNew") -> [w1027]
            shift-right: [w1024] -> _
            shift-left: 0.0 ("xNew") -> [w1026]
            shift-right: [w1023] -> _
            shift-left: 0.0 ("yNew") -> [w1025]
            tunnel: [w1031] -> w983 mode=indexing
            tunnel: [w1030] -> _ mode=indexing
            tunnel: [w1029] -> w987 mode=indexing
            tunnel: [w1028] -> w988 mode=indexing
            tunnel: [w1005] -> w979 mode=indexing
            tunnel: [w1004] -> w978 mode=indexing
            i -> [w1088]
            stop <- w1071 stop-if-true
            (unwired) 0
            w1050 = 1.0 ("y")
            (unwired) cluster{dbl, dbl, dbl} {0.2, 1e-06, 10000.0}
            w1069 = 1.0 ("y")
            (unwired) cluster{dbl, dbl, dbl} {0.2, 1e-06, 10000.0}
            # "y"
            # "y"
            # "x"
            # "x"
            # "theta"
            # "desired"
            # "phiL now"
            # "phiR now"
            # "last desired phiL"
            # "last  desired phiR"
            n75 = node-c288() -> ()  [unwired: 1 in, 1 out]
            n76 = Divide(x=w1088, y=1000) -> (x/y=w1030:dbl)
            n77 = mathscript code="a1 = (Vmax-0)/(t1-0);\na2 = (0-Vmax)/(t3-t2);\na3 = (Vmax-0)/(t7-t6); \na4 = (0-Vmax)/(t9-t8);\nb1 = (thetaDotmax-0)/(t4-t3);\nb2 = (0-thetaDotmax)/(t6-t5); \nl = 0.232;\nr = 0.037;\n\nif (t>0 && t<=t1)\nv = 0 + a1 * t;\nthetaDot = 0\nelseif (t>t1 && t<=t2)\nv = Vmax;\nthetaDot = 0\nelseif (t>t2 && t<=t3)\nv = Vmax + a2 * (t - t2);\nthetaDot = 0\nelseif (t>t3 && t<=t4)\nv = 0;\nthetaDot = 0 + b1 * (t - t3);\nelseif (t>t4 && t<=t5)\nv = 0;\nthetaDot = thetaDotmax;\nelseif (t>t5 && t<=t6)\nv = 0;\nthetaDot=  thetaDotmax + b2 * (t - t5);\nelseif (t>t6 && t<=t7)\nv = 0 + a3 *(t - t6);\nthetaDot = 0\nelseif (t>t7 && t<=t8)\nv = Vmax;\nthetaDot = 0\nelseif (t>t8 && t<=t9)\nv = Vmax + a4 * (t - t8);\nthetaDot = 0\nelse\nv = 0;\nthetaDot = 0;\nend\n\n% wheel angular velocity \nomegaR = 1 / r * (v+l*thetaDot);\nomegaL = 1 / r * (v-l*thetaDot);\nomegaR = omegaR/pi*180;\nomegaL = omegaL/pi*180;\n% wheel angular displacement\nphiR = lastPhiR + omegaR * dt;\nphiL = lastPhiL + omegaL * dt;\n%  car steering angular displacement\nthetaNew = thetaOrg + thetaDot * dt;\n%  car displacement in x&y direction\nxDot = cos(thetaNew/180*pi) * r / 2 * (omegaR+omegaL);\nxNew = xOrg + xDot * dt;\nyDot = sin(thetaNew/180*pi) * r / 2 * (omegaR+omegaL);\nyNew = xOrg + yDot * dt;\n\n% v and theta has calculated already here"("t1"="t1 case2", "t2"="t2 case2", "t3"="t3 case2", "Vmax"="Vmax (m/s) case2", "t"=w1030, "lastPhiR"=w1086, "lastPhiL"=w1085, "dt"=w994, "thetaDot"=0, "thetaOrg"=w1027, "xOrg"=w1026, "yOrg"=w1025, "t4"="t4 case2", "t5"="t5 case2", "t6"="t6 case2", "t7"="t7 case2", "t8"="t8 case2", "t9"="t9 case2", "thetaDotmax"="thetaDotmax case2") -> ("omegaR"=w1034:dbl, "omegaL"=w1033:dbl, "phiL"=w1041:dbl, "phiR"=w1040:dbl, "thetaNew"=w1022:dbl, "xNew"=w1024:dbl, "yNew"=w1023:dbl, "thetaDot"=→"thetaDot case2":dbl)  [unwired: 1 in, 2 out]
            n78 = xnode "Encoder L 2"("Reset Counter"=FALSE) -> ("Counter Value"=w1064:i32)  [unwired: 1 in, 3 out]
            n79 = xnode "Encoder R 2"("Reset Counter"=FALSE) -> ("Counter Value"=w1083:i32)  [unwired: 1 in, 3 out]
            n80 = Divide(x=w1064, y=32000) -> (x/y=w1065:dbl)
            n81 = Divide(x=w1083, y=32000) -> (x/y=w1084:dbl)
            n82 = Multiply(x=360.0, y=w1065) -> (x*y=w1037:dbl)
            n83 = Subtract(x=w1037, y=w1038) -> (x-y=w1039:dbl)
            n84 = Divide(x=w1039, y=w994) -> (x/y=w1035:dbl)
            n85 = Multiply(x=360.0, y=w1084) -> (x*y=w1043:dbl)
            n86 = Subtract(x=w1043, y=w1044) -> (x-y=w1042:dbl)
            n87 = Divide(x=1.0, y=w994) -> (x/y=w993:dbl)
            n88 = call "PID_controller.vi"("Time Period"=w993, "state(k-1)"=w1045, "Gain"="L Gain case2", "variable"=w1037, "set point"=w1041) -> ("PID gain"=w1048:dbl, "state(k)"=w1046:dbl[])
            n89 = Divide(x=1.0, y=w994) -> (x/y=w996:dbl)
            n90 = call "PID_controller.vi"("Time Period"=w996, "state(k-1)"=w1080, "Gain"="R Gain case2", "variable"=w1043, "set point"=w1040) -> ("PID gain"=w1067:dbl, "state(k)"=w1079:dbl[])
            n91 = Divide(x=w1042, y=w994) -> (x/y=w1036:dbl)
            n92 = Absolute Value(x=w1048) -> (abs(x)=w1049:dbl)
            n93 = Absolute Value(x=w1067) -> (abs(x)=w1068:dbl)
            n94 = Greater?(x=w1048, y=0.0) -> (0:w1056:bool)
            n95 = Greater?(x=w1067, y=0.0) -> (0:w1075:bool)
            n96 = Greater?(x=w1049, y=w1050) -> (0:w1051:bool)
            n97 = Bundle(w1036, "omegaR"=w1034) -> (→"phi R now, desired case2":cluster{dbl, "omegaR":dbl})  [unwired: 1 in]
            n98 = Not(x=w1056) -> (.not. x?=w1057:bool)
            n99 = Greater?(x=w1068, y=w1069) -> (0:w1070:bool)
            n100 = Not(x=w1075) -> (.not. x?=w1076:bool)
            n101 = Not(x=w1057) -> (.not. x?=w1054:bool)
            n102 = Select(t=w1050, s=w1051, f=w1049) -> (s? t:f=w1047:dbl)
            "Duty L case2" <- w1047
            n103 = Not(x="stop case2") -> (.not. x?=w1053:bool)
            n104 = Not(x=w1076) -> (.not. x?=w1073:bool)
            n105 = Select(t=w1069, s=w1070, f=w1068) -> (s? t:f=w1066:dbl)
            n106 = Not(x="stop case2") -> (.not. x?=w1072:bool)
            n107 = And(x=w1057, y=w1053) -> (x .and. y?=w1060:bool)
            n108 = And(x=w1054, y=w1053) -> (x .and. y?=w1058:bool)
            n109 = And(x=w1076, y=w1072) -> (x .and. y?=w1078:bool)
            n110 = And(x=w1073, y=w1072) -> (x .and. y?=w1077:bool)
            n111 = Not(x=w1072) -> (.not. x?=w1071:bool)
            n112 = Not(x=w1060) -> (.not. x?=w1061:bool)
            n113 = Not(x=w1058) -> (.not. x?=w1059:bool)
            n114 = xnode "PWM L 2"("Duty Cycle"=w1047, "Frequency [Hz]"="Frequency L [Hz] case2") -> ()  [unwired: 1 in, 1 out]
            n115 = Not(x=w1078) -> (.not. x?=w1001:bool)
            n116 = Not(x=w1077) -> (.not. x?=w1000:bool)
            n117 = xnode "PWM R 2"("Duty Cycle"=w1066, "Frequency [Hz]"="Frequency R [Hz] case2") -> ()  [unwired: 1 in, 1 out]
            n118 = xnode "DIR L 2"("A/DIO0 (Pin 11)"=w1061, "A/DIO1 (Pin 13)"=w1059) -> ()  [unwired: 1 in, 1 out]
            n119 = Bundle(w1035, "omegaL"=w1033) -> (→"phi L now, desired case2":cluster{dbl, "omegaL":dbl})  [unwired: 1 in]
            n120 = xnode "DIR R 2"("B/DIO0 (Pin 11)"=w1001, "B/DIO1 (Pin 13)"=w1000) -> ()  [unwired: 1 in, 1 out]
            n121 = mathscript code="l = 0.232;\nr = 0.037;\n\nactCarV = 1 / 2 * r * ( actOmegaR + actOmegaL) / 180 * pi;;\nactCarOmega = 1 / 2 / l * r * ( actOmegaR - actOmegaL) / 180 * pi;;\n\ndesCarV = 1 / 2 * r * ( desOmegaR + desOmegaL) / 180 * pi;\ndesCarOmega = 1 / 2 / l * r * ( desOmegaR - desOmegaL) / 180 * pi;\n\n% desXDot = cos(theta)*desCarV"("desOmegaR"=w1034, "desOmegaL"=w1033, "actOmegaR"=w1036, "actOmegaL"=w1035) -> ("actCarOmega"=w1005:dbl, "desCarOmega"=w1004:dbl, "actCarV"=w1028:dbl, "desCarV"=w1029:dbl)  [unwired: 1 in, 1 out]
            n122 = Build Array(w1024, w1023) -> (w1031:dbl[])
            n123 = Bundle("actCarOmega"=w1005, "desCarOmega"=w1004) -> (→"CarOmega case2":cluster{"actCarOmega":dbl, "desCarOmega":dbl})  [unwired: 1 in]
            n124 = Bundle("actCarV"=w1028, "desCarV"=w1029) -> (→"CarV case2":cluster{"actCarV":dbl, "desCarV":dbl})  [unwired: 1 in]
            n125 = node-c288() -> ()  [unwired: 1 in, 1 out]
          }
          "XY Graph case2" <- w983
          n126 = node-c288(w989) -> ()  [unwired: 1 out]
          n127 = call "Convert to Dynamic Data3"("Array"=w988) -> ("Dynamic Data Type"=w986:dynamicdata)  [unwired: 3 in]
          n128 = call "Convert to Dynamic Data4"("Array"=w987) -> ("Dynamic Data Type"=w985:dynamicdata)  [unwired: 3 in]
          n129 = call "Convert to Dynamic Data5"("Array"=w979) -> ("Dynamic Data Type"=w982:dynamicdata)  [unwired: 3 in]
          n130 = call "Convert to Dynamic Data6"("Array"=w978) -> ("Dynamic Data Type"=w981:dynamicdata)  [unwired: 3 in]
          n131 = Merge Signals(w986, w985) -> (→"carVTest Chart case2":dynamicdata)
          n132 = Merge Signals(w982, w981) -> (→"carOmegaTest case2":dynamicdata)
        }
        frame "Page 3" {
          w2215 = dbl[] [] ("state(k)")
          w2218 = i64 1 ("Period")
          n133 = Divide(x=w2218, y=i64 1000) -> (x/y=w2216:dbl)
          n134 = node-c288(w2218) -> (w2231:T16)  [unwired: 3 in]
          n135 = timed-loop {
            timing: w2231 -> [_]
            timing-out: [_] -> w2230
            shift-right: [w2278] -> _
            shift-left: 0.0 ("phiR") -> [w2325]
            shift-right: [w2279] -> _
            shift-left: 0.0 ("phiL") -> [w2324]
            tunnel: w2216 -> [w2233]
            shift-right: [w2318] -> _
            shift-left: w2215 -> [w2319]
            shift-right: [w2284] -> _
            shift-left: w2215 -> [w2283]
            shift-right: [w2281] -> _
            shift-left: _ -> [w2282]
            shift-right: [w2275] -> _
            shift-left: _ -> [w2276]
            shift-right: [w2260] -> _
            shift-left: 0.0 ("thetaNew") -> [w2265]
            shift-right: [w2262] -> _
            shift-left: 0.0 ("xNew") -> [w2264]
            shift-right: [w2261] -> _
            shift-left: 0.0 ("yNew") -> [w2263]
            tunnel: [w2269] -> w2224 mode=indexing
            tunnel: [w2267] -> w2220 mode=indexing
            tunnel: [w2266] -> w2219 mode=indexing
            tunnel: [w2245] -> w2228 mode=indexing
            tunnel: [w2244] -> w2229 mode=indexing
            i -> [w2327]
            stop <- w2310 stop-if-true
            w2288 = 1.0 ("y")
            (unwired) cluster{dbl, dbl, dbl} {0.2, 1e-06, 10000.0}
            w2307 = 1.0 ("y")
            (unwired) cluster{dbl, dbl, dbl} {0.2, 1e-06, 10000.0}
            # "y"
            # "y"
            # "x"
            # "x"
            # "theta"
            # "desired"
            # "phiL now"
            # "phiR now"
            # "last desired phiL"
            # "last  desired phiR"
            n136 = node-c288() -> ()  [unwired: 1 in, 1 out]
            n137 = Divide(x=w2327, y=1000) -> (x/y=w2268:dbl)
            n138 = mathscript code="a1 = (Vmax-0)/(t1-0);\na2 = (0-Vmax)/(t7-t6);\nb1 = (thetaDotmax-0)/(t3-t2);\nb2 = (0-thetaDotmax)/(t5-t4); \nl = 0.232;\nr = 0.037;\n\nif (t>0 && t<=t1)\nv = 0 + a1 * t;\nthetaDot = 0;\nelseif (t>t1 && t<=t2)\nv = Vmax;\nthetaDot = 0;\nelseif (t>t2 && t<=t3)\nv = Vmax;\nthetaDot = 0 + b1 * (t - t2);\nelseif (t>t3 && t<=t4)\nv = Vmax;\nthetaDot = thetaDotmax;\nelseif (t>t4 && t<=t5)\nv = Vmax;\nthetaDot=  thetaDotmax + b2 * (t - t4);\nelseif (t>t5 && t<=t6)\nv = Vmax;\nthetaDot = 0;\nelseif (t>t6 && t<=t7)\nv = Vmax + a2 * (t - t6);\nthetaDot = 0;\nelse\nv = 0;\nthetaDot = 0;\nend\n\n% wheel angular velocity \nomegaR = 1 / r * (v+l*thetaDot);\nomegaL = 1 / r * (v-l*thetaDot);\nomegaR = omegaR/pi*180;\nomegaL = omegaL/pi*180;\n% wheel angular displacement\nphiR = lastPhiR + omegaR * dt;\nphiL = lastPhiL + omegaL * dt;\n%  car steering angular displacement\nthetaNew = thetaOrg + thetaDot * dt;\n%  car displacement in x&y direction\nxDot = cos(thetaNew/180*pi) * r / 2 * (omegaR+omegaL);\nxNew = xOrg + xDot * dt;\nyDot = sin(thetaNew/180*pi) * r / 2 * (omegaR+omegaL);\nyNew = xOrg + yDot * dt;"("t1"="t1 case3", "t2"="t2 case3", "t3"="t3 case3", "Vmax"="Vmax (m/s) case3", "t"=w2268, "lastPhiR"=w2325, "lastPhiL"=w2324, "dt"=w2233, "thetaDot"=0, "thetaOrg"=w2265, "xOrg"=w2264, "yOrg"=w2263, "t4"="t4 case3", "t5"="t5 case3", "t6"="t6 case3", "t7"="t7 case3", "thetaDotmax"="thetaDotmax case3") -> ("omegaR"=w2272:dbl, "omegaL"=w2271:dbl, "phiL"=w2279:dbl, "phiR"=w2278:dbl, "thetaNew"=w2260:dbl, "xNew"=w2262:dbl, "yNew"=w2261:dbl, "thetaDot"=→"thetaDot case3":dbl)  [unwired: 1 in, 2 out]
            n139 = xnode "Encoder L 3"("Reset Counter"=FALSE) -> ("Counter Value"=w2302:i32)  [unwired: 1 in, 3 out]
            n140 = xnode "Encoder R 3"("Reset Counter"=FALSE) -> ("Counter Value"=w2322:i32)  [unwired: 1 in, 3 out]
            n141 = Divide(x=w2302, y=32000) -> (x/y=w2303:dbl)
            n142 = Divide(x=w2322, y=32000) -> (x/y=w2323:dbl)
            n143 = Multiply(x=360.0, y=w2303) -> (x*y=w2275:dbl)
            n144 = Subtract(x=w2275, y=w2276) -> (x-y=w2277:dbl)
            n145 = Divide(x=w2277, y=w2233) -> (x/y=w2273:dbl)
            n146 = Multiply(x=360.0, y=w2323) -> (x*y=w2281:dbl)
            n147 = Divide(x=1.0, y=w2233) -> (x/y=w2232:dbl)
            n148 = Subtract(x=w2281, y=w2282) -> (x-y=w2280:dbl)
            n149 = call "PID_controller.vi"("Time Period"=w2232, "state(k-1)"=w2283, "Gain"="L Gain case3", "variable"=w2275, "set point"=w2279) -> ("PID gain"=w2286:dbl, "state(k)"=w2284:dbl[])
            n150 = Divide(x=1.0, y=w2233) -> (x/y=w2235:dbl)
            n151 = call "PID_controller.vi"("Time Period"=w2235, "state(k-1)"=w2319, "Gain"="R Gain case3", "variable"=w2281, "set point"=w2278) -> ("PID gain"=w2305:dbl, "state(k)"=w2318:dbl[])
            n152 = Divide(x=w2280, y=w2233) -> (x/y=w2274:dbl)
            n153 = Absolute Value(x=w2286) -> (abs(x)=w2287:dbl)
            n154 = Absolute Value(x=w2305) -> (abs(x)=w2306:dbl)
            n155 = Greater?(x=w2286, y=0.0) -> (0:w2294:bool)
            n156 = Greater?(x=w2305, y=0.0) -> (0:w2314:bool)
            n157 = Greater?(x=w2287, y=w2288) -> (0:w2289:bool)
            n158 = Bundle(w2274, "omegaR"=w2272) -> (→"phi R now, desired case3":cluster{dbl, "omegaR":dbl})  [unwired: 1 in]
            n159 = Not(x=w2294) -> (.not. x?=w2295:bool)
            n160 = Greater?(x=w2306, y=w2307) -> (0:w2308:bool)
            n161 = Not(x=w2314) -> (.not. x?=w2315:bool)
            n162 = Not(x=w2295) -> (.not. x?=w2292:bool)
            n163 = Select(t=w2288, s=w2289, f=w2287) -> (s? t:f=w2285:dbl)
            "Duty L case3" <- w2285
            n164 = Not(x="stop case3") -> (.not. x?=w2291:bool)
            n165 = Not(x=w2315) -> (.not. x?=w2312:bool)
            n166 = Select(t=w2307, s=w2308, f=w2306) -> (s? t:f=w2304:dbl)
            "Duty R case3" <- w2304
            n167 = Not(x="stop case3") -> (.not. x?=w2311:bool)
            n168 = And(x=w2295, y=w2291) -> (x .and. y?=w2298:bool)
            n169 = And(x=w2292, y=w2291) -> (x .and. y?=w2296:bool)
            n170 = And(x=w2315, y=w2311) -> (x .and. y?=w2317:bool)
            n171 = And(x=w2312, y=w2311) -> (x .and. y?=w2316:bool)
            n172 = Not(x=w2311) -> (.not. x?=w2310:bool)
            n173 = Not(x=w2298) -> (.not. x?=w2299:bool)
            n174 = Not(x=w2296) -> (.not. x?=w2297:bool)
            n175 = xnode "PWM L 3"("Duty Cycle"=w2285, "Frequency [Hz]"="Frequency L [Hz] case3") -> ()  [unwired: 1 in, 1 out]
            n176 = Not(x=w2317) -> (.not. x?=w2242:bool)
            n177 = Not(x=w2316) -> (.not. x?=w2241:bool)
            n178 = xnode "PWM R 3"("Duty Cycle"=w2304, "Frequency [Hz]"="Frequency R [Hz] case3") -> ()  [unwired: 1 in, 1 out]
            n179 = Bundle(w2273, "omegaL"=w2271) -> (→"phi L now, desired case3":cluster{dbl, "omegaL":dbl})  [unwired: 1 in]
            n180 = xnode "DIR L 3"("A/DIO0 (Pin 11)"=w2299, "A/DIO1 (Pin 13)"=w2297) -> ()  [unwired: 1 in, 1 out]
            n181 = xnode "DIR R 3"("B/DIO0 (Pin 11)"=w2242, "B/DIO1 (Pin 13)"=w2241) -> ()  [unwired: 1 in, 1 out]
            n182 = mathscript code="l = 0.232;\nr = 0.037;\n\nactCarV = 1 / 2 * r * ( actOmegaR + actOmegaL) / 180 * pi;\nactCarOmega = 1 / 2 / l * r * ( actOmegaR - actOmegaL) / 180 * pi;\n\ndesCarV = 1 / 2 * r * ( desOmegaR + desOmegaL) / 180 * pi;\ndesCarOmega = 1 / 2 / l * r * ( desOmegaR - desOmegaL) / 180 * pi;\n\n% desXDot = cos(theta)*desCarV"("desOmegaR"=w2272, "desOmegaL"=w2271, "actOmegaR"=w2274, "actOmegaL"=w2273) -> ("actCarOmega"=w2245:dbl, "desCarOmega"=w2244:dbl, "actCarV"=w2266:dbl, "desCarV"=w2267:dbl)  [unwired: 1 in, 1 out]
            n183 = Build Array(w2262, w2261) -> (w2269:dbl[])
            n184 = Bundle("actCarOmega"=w2245, "desCarOmega"=w2244) -> (→"CarOmega case3":cluster{"actCarOmega":dbl, "desCarOmega":dbl})  [unwired: 1 in]
            n185 = Bundle("actCarV"=w2266, "desCarV"=w2267) -> (→"CarV case3":cluster{"actCarV":dbl, "desCarV":dbl})  [unwired: 1 in]
            n186 = node-c288() -> ()  [unwired: 1 in, 1 out]
          }
          "XY Graph case3" <- w2224
          n187 = node-c288(w2230) -> ()  [unwired: 1 out]
          n188 = call "Convert to Dynamic Data7"("Array"=w2219) -> ("Dynamic Data Type"=w2221:dynamicdata)  [unwired: 3 in]
          n189 = call "Convert to Dynamic Data8"("Array"=w2220) -> ("Dynamic Data Type"=w2222:dynamicdata)  [unwired: 3 in]
          n190 = call "Convert to Dynamic Data9"("Array"=w2228) -> ("Dynamic Data Type"=w2225:dynamicdata)  [unwired: 3 in]
          n191 = call "Convert to Dynamic Data10"("Array"=w2229) -> ("Dynamic Data Type"=w2226:dynamicdata)  [unwired: 3 in]
          n192 = Merge Signals(w2221, w2222) -> (→"carV Chart case3":dynamicdata)
          n193 = Merge Signals(w2225, w2226) -> (→"carOmega Chart case3":dynamicdata)
        }
      }
    }
  }
